vi "Clear FF buffers.vi"(8 "error in (no error)":errorcluster, 10 "Force":bool, 11 "FpgaRef5785 in":refnum<class "FpgaRef5782.lvclass">) -> (0 "error out":errorcluster, 3 "FpgaRef5785 out":refnum<class "FpgaRef5782.lvclass">)   [LabVIEW 2025, in "FpgaRef5782.lvclass"]
uses:
  FpgaRef5782.lvclass
  FpgaRef5782.lvclass/FpgaRef5782.ctl
  <vilib>/rvi/interface/nirviReadWriteControl/nirviReadWriteControl.xnode
  <vilib>/rvi/interface/Simulation/niFpgaSimulationCallBeginRW.vi
  <vilib>/rvi/errors/niLvFpgaAdjustHostInterfaceError.vi
  <userlib>/_OpenG.lib/time/time.llb/openg_time.lvlib
  5782 FPGA ref.ctl
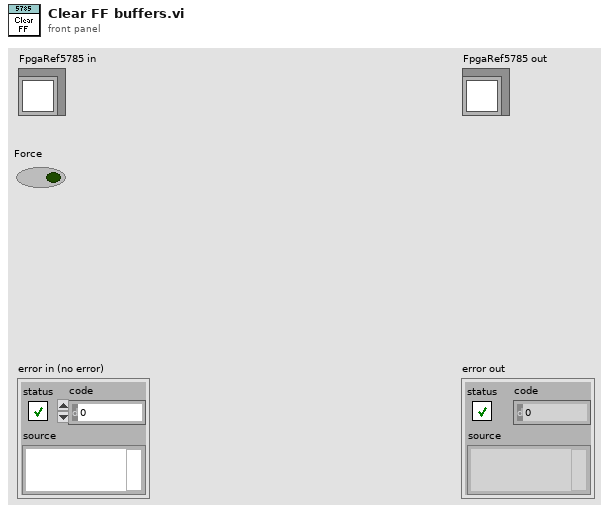
[diagram p1: front panel]
types:
  T1 = typedef "5782 FPGA ref.ctl" = refnum<k20>
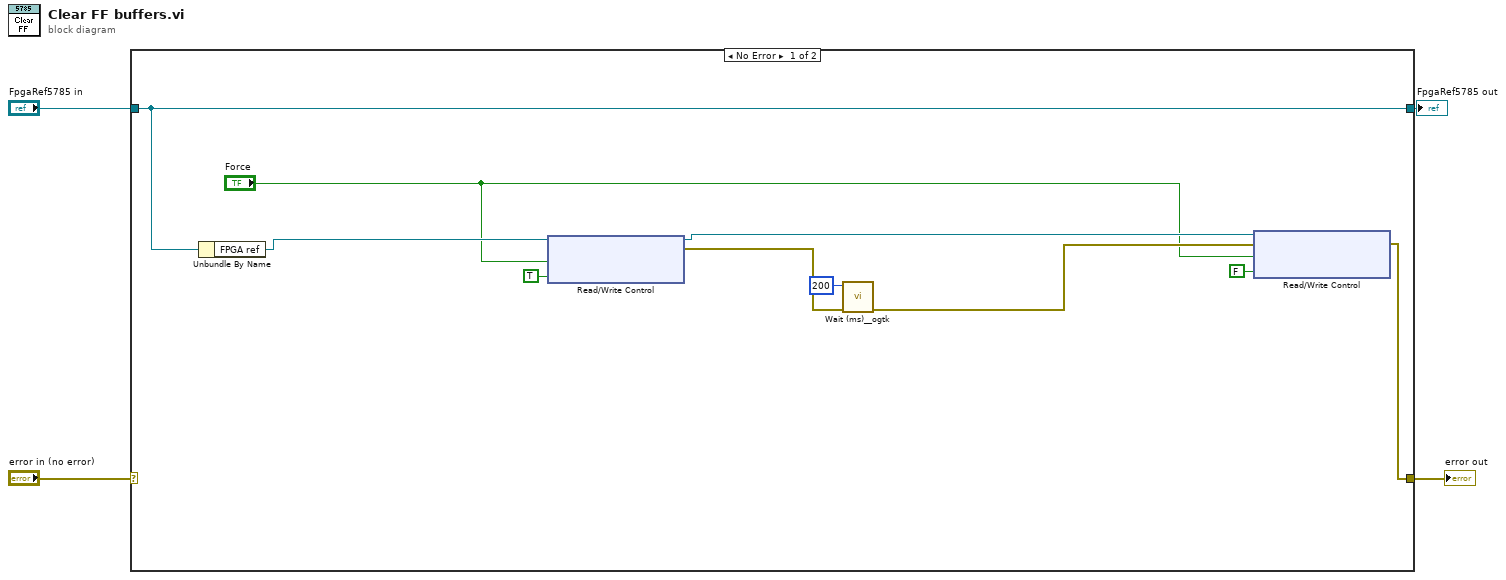
[diagram p0: block diagram]
diagram:
  n1 = case shown="No Error" "error in (no error)" {
    selector: "error in (no error)" -> [_ w16]
    tunnel: [w9 w16] -> w3
    tunnel: [w10 w15] -> w1
    tunnel: "FpgaRef5785 in" -> [w10 w15]
    frame No Error {
      n2 = Unbundle By Name(w10) -> ("FPGA ref"=w7:T1)
      n3 = xnode "Read/Write Control"("FPGA VI Reference In"=w7, "FF buffers manual"="Force", "Clear feedback buffers"=TRUE ("Load FF")) -> ("FPGA VI Reference Out"=w6:T1, "error out"=w13:errorcluster)  [unwired: 1 in]
      n4 = call <userlib>:"Wait (ms)__ogtk.vi"("error in (no error)"=w13, "milliseconds to wait"=u32 200) -> ("error out"=w8:errorcluster)  [unwired: 8 in, 1 out]
      n5 = xnode "Read/Write Control"("FPGA VI Reference In"=w6, "error in"=w8, "FF buffers manual"="Force", "Clear feedback buffers"=FALSE ("Load FF")) -> ("error out"=w9:errorcluster)  [unwired: 1 out]
    }
    frame Error {
    }
  }
  "error out" <- w3
  "FpgaRef5785 out" <- w1
